vi "Push Backup to DB.vi"(7 "Backup lines at a time":i32=1, 10 "Path to backup file":path, 11 "Data.PG":refnum<class "LV-Data.PGSQL.lvclass">) -> ()   [LabVIEW 2019, in "LV-Data.PGSQL.lvclass"]
uses:
  LV-Data.PGSQL.lvclass
  Typedefs/Time.Datatype--enum.ctl
  LV-Data.PGSQL.lvclass/LV-Data.PGSQL.ctl
  <vilib>/JDP Science/PostgreSQL Library/Connection/Execute Command (No results).vi
  <vilib>/JDP Science/PostgreSQL Library/Connection/Execute Command (Result).vi
  <vilib>/JDP Science/PostgreSQL Library/Result/Clear.vi
  <vilib>/JDP Science/PostgreSQL Library/Connection/PQ Connection.lvclass
panel:
  out "Success?":bool
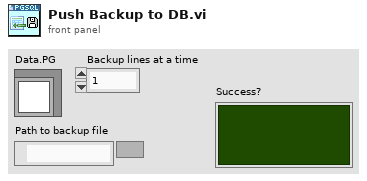
[diagram p1: front panel]
types:
  T1 = typedef "LV-Data.PGSQL.lvclass/Time.Datatype--enum.ctl" = enum16{"timestamp without time zone", "timestamp with time zone"}
  T2 = enum16{"open", "replace", "create", "open or create", "replace or create", "replace or create with confirmation"}
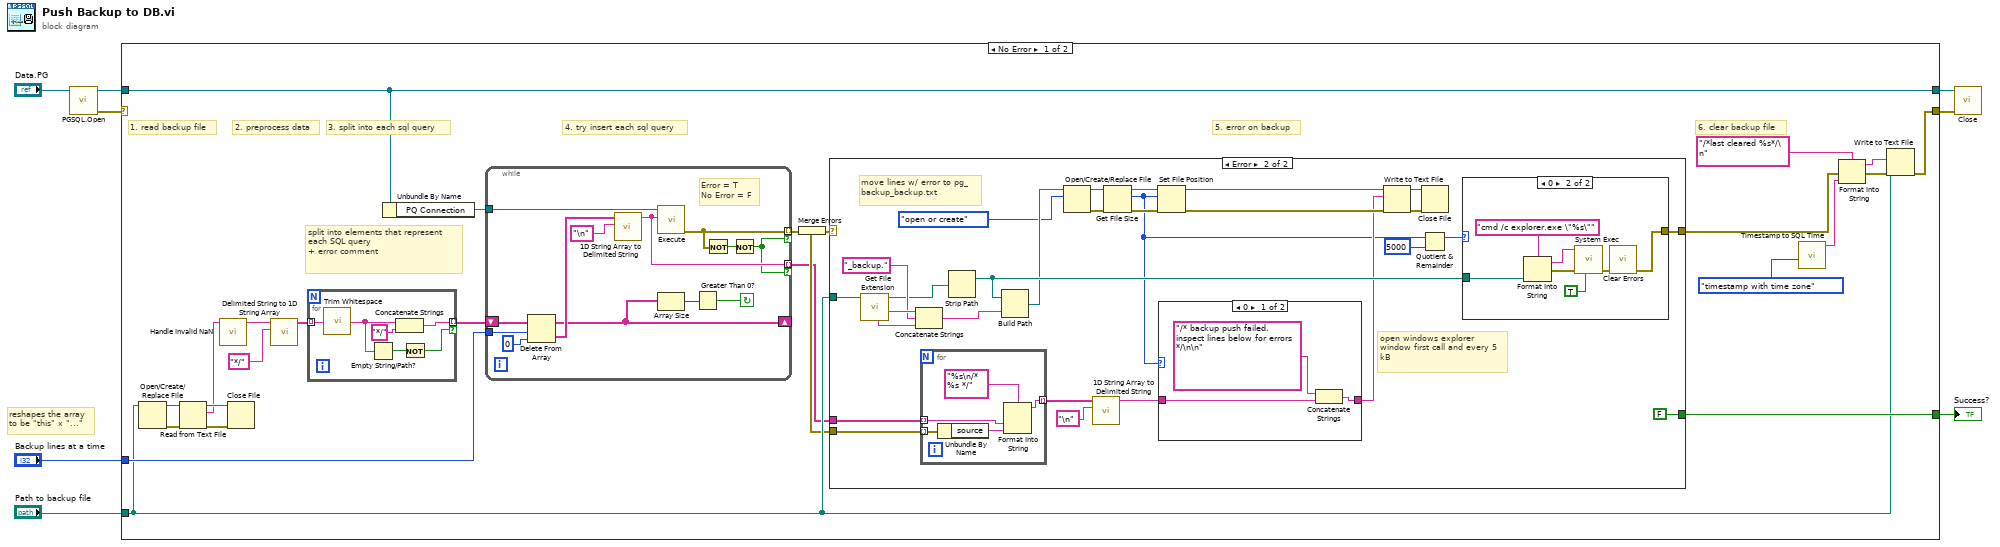
[diagram p0: block diagram]
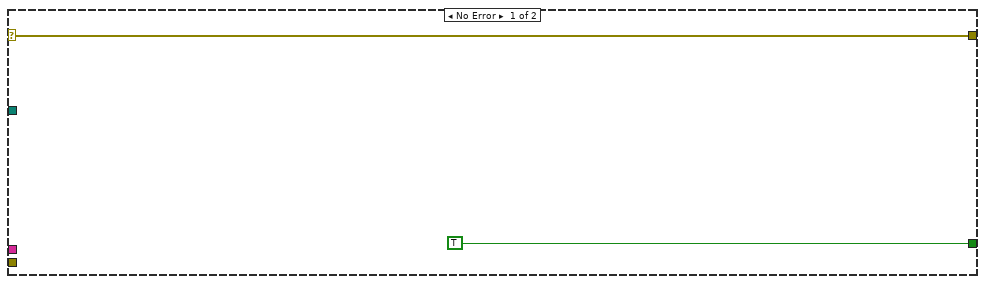
[diagram p2: hidden frame]
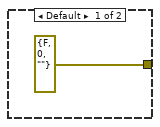
[diagram p4: hidden frame]
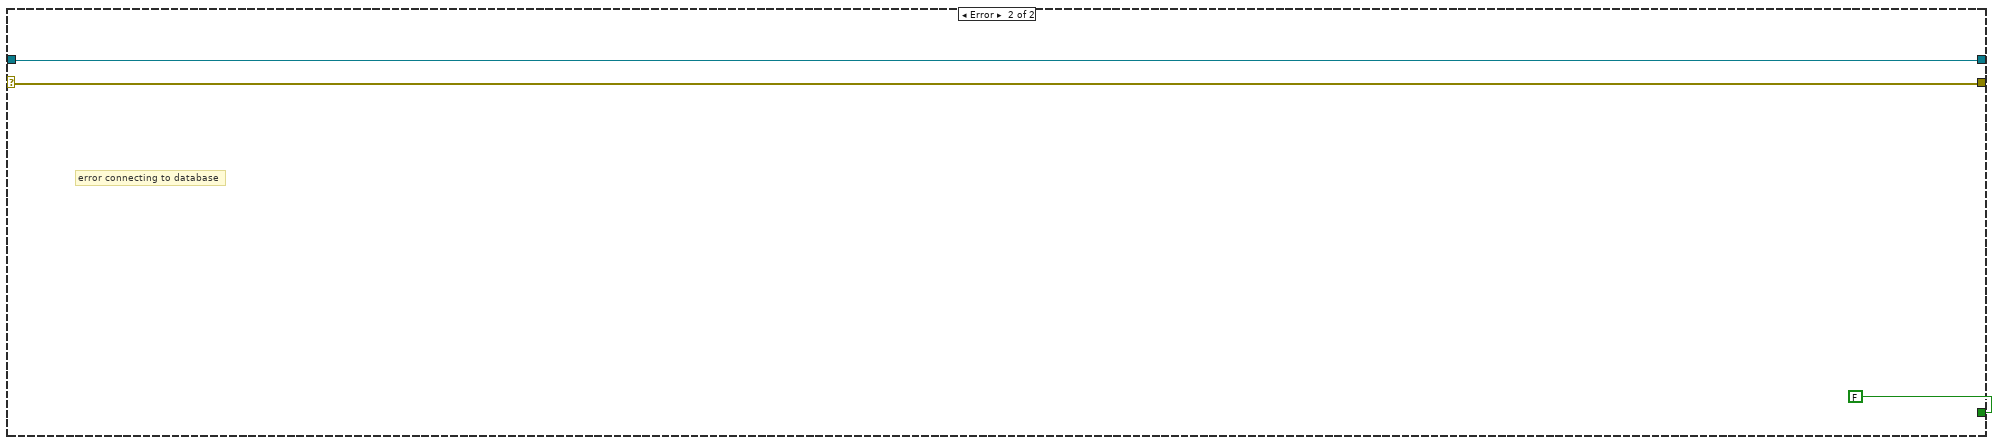
[diagram p5: hidden frame]
diagram:
  # "reshapes the array\nto be \"this\" x \"...\""
  n1 = call "PGSQL.Open.vi"("Data.PG in"="Data.PG") -> ("error out"=w3:errorcluster, "Data.PG out"=w7:refnum<class "LV-Data.PGSQL.lvclass">)  [unwired: 9 in]
  n2 = case shown="No Error" w3 {
    selector: w3 -> [_ w100]
    tunnel: w7 -> [w15 w101]
    tunnel: "Backup lines at a time" -> [w30 _]
    tunnel: [w14 FALSE] -> w5
    tunnel: [w9 w100] -> w4
    tunnel: "Path to backup file" -> [w13 _]
    tunnel: [w15 w101] -> w1
    frame No Error {
      # "6. clear backup file"
      # "5. error on backup"
      # "4. try insert each sql query"
      # "3. split into each sql query"
      # "2. preprocess data"
      # "1. read backup file"
      # "split into elements that represent each SQL query\n+ error comment"
      n3 = Open/Create/Replace File(file path (use dialog)=w13) -> (refnum out=w31:refnum<file>, error out=w32:errorcluster)  [unwired: 5 in, 1 out]
      n4 = Read from Text File(file (use dialog)=w31, error in=w32) -> (refnum out=w29:refnum<file>, text=w27:string, error out=w28:errorcluster)  [unwired: 2 in, 1 out]
      n5 = call "Handle Invalid NaN.vi"("String"=w27) -> ("result string"=w22:string)  [unwired: 10 in]
      n6 = Close File(refnum=w29, error in=w28) -> ()  [unwired: 2 out]
      n7 = call <vilib>:"Delimited String to 1D String Array.vi"("delimiter"="*/", "delimited string"=w22) -> ("string array"=w24:string[])  [unwired: 9 in]
      n8 = for {
        tunnel: w24 -> [w84] mode=indexing
        tunnel: [w85] -> w23 mode=indexing if=w80
        n9 = call <vilib>:"Trim Whitespace.vi"("string"=w84) -> ("trimmed string"=w83:string)  [unwired: 1 in]
        n10 = Empty String/Path?(string/path=w83) -> (empty?=w81:bool)
        n11 = Concatenate Strings(w83, "*/" ("string")) -> (w85:string)
        n12 = Not(x=w81) -> (.not. x?=w80:bool)
      }
      n13 = Unbundle By Name(w15) -> ("PQ Connection"=w26:refnum<class "PQ Connection.lvclass">)
      n14 = while {
        tunnel: w26 -> [w96]
        shift-right: [w90] -> _
        shift-left: w23 -> [w95]
        tunnel: [w88] -> w12 mode=indexing if=w86
        tunnel: w30 -> [w92]
        tunnel: [w89] -> w11 mode=indexing if=w86
        stop <- w91 continue-if-true
        # "Error = T\nNo Error = F"
        n15 = Delete From Array(array=w95, length=w92, index=0) -> (deleted portion=w94:string[], array with subset deleted=w90:string[])
        n16 = call <vilib>:"1D String Array to Delimited String.vi"("delimiter"="\n", "string array"=w94) -> ("delimited string"=w89:string)  [unwired: 9 in]
        n17 = call-poly <vilib>:"Execute.vi"("SQL"=w89, "PQ Connection in"=w96) -> ("error out"=w88:errorcluster)  [unwired: 8 in, 1 out]
        n18 = Array Size(array=w90) -> (size(s)=w93:i32)
        n19 = Greater Than 0?(x=w93) -> (x > 0?=w91:bool)
        n20 = Not(x=w88) -> (.not. x?=w87:bool)
        n21 = Not(x=w87) -> (.not. x?=w86:bool)
      }
      n22 = Merge Errors(w12) -> (w16:errorcluster)
      n23 = case shown="Error" w16 {
        selector: w16 -> [w33 _]
        tunnel: w13 -> [_ w53]
        tunnel: [TRUE FALSE] -> w14
        tunnel: w11 -> [_ w41]
        tunnel: [w33 w44] -> w17
        tunnel: w12 -> [_ w42]
        frame No Error {
        }
        frame Error {
          # "open windows explorer window first call and every 5 kB"
          # "move lines w/ error to pg_backup_backup.txt"
          n24 = call <vilib>:"Get File Extension.vi"("file"=w53) -> ("filename without extension"=w59:string, "dup file"=w54:path, "unmodified file extension"=w58:string)  [unwired: 6 in, 2 out]
          n25 = Concatenate Strings(w59, "_backup." ("string"), w58) -> (w56:string)
          n26 = for {
            tunnel: w42 -> [w71] mode=indexing
            tunnel: w41 -> [w67] mode=indexing
            tunnel: [w68] -> w39 mode=indexing
            n27 = Unbundle By Name(w71) -> ("source"=w70:string)
            n28 = Format Into String(format string="%s\n/* %s */", w67, w70) -> (resulting string=w68:string)  [unwired: 2 in, 1 out]
          }
          n29 = Strip Path(path=w54) -> (stripped path=w55:path)  [unwired: 1 out]
          n30 = Build Path(base path=w55, name or relative path=w56) -> (appended path=w43:path)
          n31 = Open/Create/Replace File(file path (use dialog)=w43, operation (0:open)=T2."open or create") -> (refnum out=w46:refnum<file>, error out=w45:errorcluster)  [unwired: 4 in, 1 out]
          n32 = call <vilib>:"1D String Array to Delimited String.vi"("delimiter"="\n", "string array"=w39) -> ("delimited string"=w38:string)  [unwired: 9 in]
          n33 = Get File Size(file=w46, error in=w45) -> (refnum out=w51:refnum<file>, size (in bytes)=w35:i64, 0:w52:errorcluster)
          n34 = Set File Position(offset (in bytes) (0)=w35, refnum=w51, error in=w52) -> (refnum out=w49:refnum<file>, error out=w50:errorcluster)  [unwired: 1 in]
          n35 = case shown="0" w35 {
            tunnel: w38 -> [w65 w66]
            tunnel: [w64 w66] -> w37
            frame 0 {
              n36 = Concatenate Strings("/* backup push failed. inspect lines below for errors */\n\n" ("string"), w65) -> (w64:string)
            }
            frame Default {
            }
          }
          n37 = Write to Text File(file (use dialog)=w49, text=w37, error in=w50) -> (refnum out=w47:refnum<file>, error out=w48:errorcluster)  [unwired: 1 in, 1 out]
          n38 = Close File(refnum=w47, error in=w48) -> ()  [unwired: 2 out]
          n39 = Quotient & Remainder(x=w35, y=i64 5000) -> (x-y*floor(x/y)=w60:i64)  [unwired: 1 out]
          n40 = case shown="0" w60 {
            tunnel: w55 -> [_ w79]
            tunnel: [errorcluster {"status"=FALSE, "code"=0, "source"=""} ("error out") w78] -> w44
            frame Default {
            }
            frame 0 {
              n41 = Format Into String(format string="cmd /c explorer.exe \"%s\"", w79) -> (resulting string=w76:string, error out=w74:errorcluster)  [unwired: 2 in]
              n42 = call <vilib>:"System Exec.vi"("run minimized? (F)"=TRUE, "error in (no error)"=w74, "command line"=w76) -> ("error out"=w73:errorcluster)  [unwired: 5 in, 3 out]
              n43 = call <vilib>:"Clear Errors.vi"("error in (no error)"=w73) -> ("error out"=w78:errorcluster)  [unwired: 5 in, 1 out]
            }
          }
        }
      }
      n44 = call "Timestamp to SQL Time.vi"("Time Datatype"=Time.Datatype--enum."timestamp with time zone") -> ("date/time string"=w19:string)  [unwired: 10 in]
      n45 = Format Into String(format string="/*last cleared %s*/\n", error in=w17, w19) -> (resulting string=w20:string, error out=w21:errorcluster)  [unwired: 1 in]
      n46 = Write to Text File(file (use dialog)=w13, text=w20, error in=w21) -> (error out=w9:errorcluster)  [unwired: 1 in, 2 out]
    }
    frame Error {
      # "error connecting to database"
    }
  }
  "Success?" <- w5
  n47 = call-dynamic "Close.vi"("error in (no error)"=w4, "Data.PG in"=w1) -> ()  [unwired: 8 in, 2 out]
